vi "HookValidationA1-check0.vi"(7 "Image In":T1, 8 "中心Y":dbl, 9 "中心X":dbl, 10 "起始钩角":sgl, 11 "最接近槽角":dbl) -> (5 "Image Out":T1)   [LabVIEW 2015]
uses:
  <vilib>/vision/Image Controls.llb/IMAQ Image.ctl
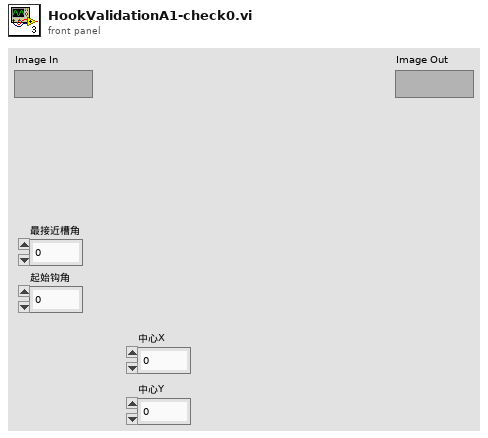
[diagram p1: front panel]
types:
  T1 = typedef "IMAQ Image.ctl" = refnum<image>
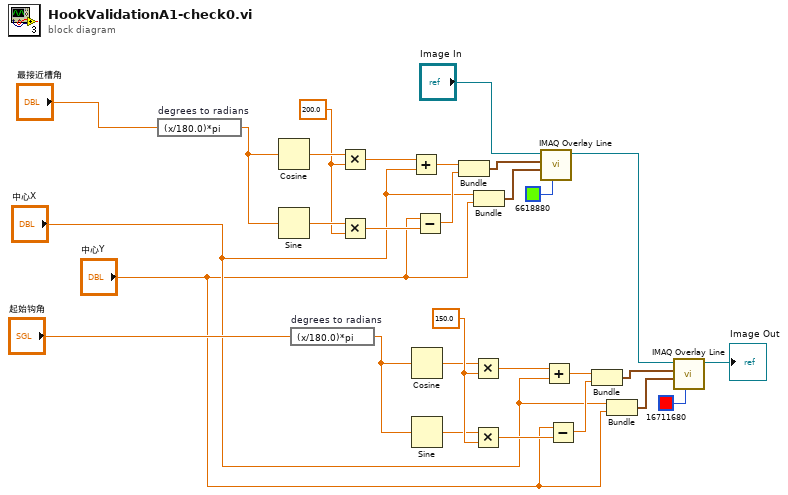
[diagram p0: block diagram]
diagram:
  w12 = 150.0
  w26 = 200.0
  n1 = expression code="(x/180.0)*pi" "degrees to radians"("最接近槽角") -> (w29:dbl)
  n2 = Cosine(x=w29) -> (cos(x)=w28:dbl)
  n3 = Sine(x=w29) -> (sin(x)=w27:dbl)
  n4 = expression code="(x/180.0)*pi" "degrees to radians"("起始钩角") -> (w9:sgl)
  n5 = Multiply(x=w28, y=w26) -> (x*y=w25:dbl)
  n6 = Multiply(x=w27, y=w26) -> (x*y=w24:dbl)
  n7 = Add(x=w25, y="中心X") -> (x+y=w21:dbl)
  n8 = Cosine(x=w9) -> (cos(x)=w10:sgl)
  n9 = Sine(x=w9) -> (sin(x)=w11:sgl)
  n10 = Subtract(x="中心Y", y=w24) -> (x-y=w22:dbl)
  n11 = Bundle(w21, w22) -> (w20:cluster{dbl, dbl})  [unwired: 1 in]
  n12 = Multiply(x=w10, y=w12) -> (x*y=w13:dbl)
  n13 = Multiply(x=w11, y=w12) -> (x*y=w14:dbl)
  n14 = Bundle("中心X"="中心X", "中心Y"="中心Y") -> (w23:cluster{"中心X":dbl, "中心Y":dbl})  [unwired: 1 in]
  n15 = call "IMAQ Overlay Line"("Color"=u32 6618880, "End Point"=w23, "Start Point"=w20, "Image"="Image In") -> ("Image Out"=w8:T1)  [unwired: 6 in, 1 out]
  n16 = Add(x=w13, y="中心X") -> (x+y=w17:dbl)
  n17 = Subtract(x="中心Y", y=w14) -> (x-y=w16:dbl)
  n18 = Bundle(w17, w16) -> (w18:cluster{dbl, dbl})  [unwired: 1 in]
  n19 = Bundle("中心X"="中心X", "中心Y"="中心Y") -> (w15:cluster{"中心X":dbl, "中心Y":dbl})  [unwired: 1 in]
  n20 = call "IMAQ Overlay Line"("Color"=u32 16711680, "End Point"=w15, "Start Point"=w18, "Image"=w8) -> ("Image Out"=→"Image Out":T1)  [unwired: 6 in, 1 out]
